vi "setFontFilters.vi"(8 "Error In":errorcluster, 10 "filters":T1 items=["AllFonts"=0, "ScalableFonts"=1, "NonScalableFonts"=2, "MonospacedFonts"=4, "ProportionalFonts"=8], 11 "QFontComboBox In":refnum<class "QFontComboBox.lvclass">) -> (0 "Error Out":errorcluster, 3 "QFontComboBox Out":refnum<class "QFontComboBox.lvclass">)   [LabVIEW 2014, in "QFontComboBox.lvclass"]
doc: "LabVIEW-specific documentation is not yet available. See <b>https://doc.qt.io/qt-5/qfontcombobox.html#setFontFilters</b>"
uses:
  QFontComboBox.lvclass
  FontFilter.ctl
  LQ Core/LQIdentity/LQIdentity.lvclass/LQIdentity.ctl
  LQ Core/LQ Core.lvlib
  LQ Core/LQIdentity/LQIdentity.lvclass
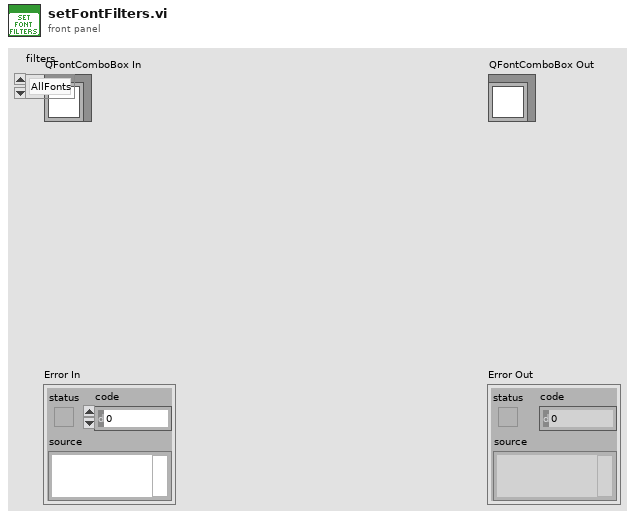
[diagram p1: front panel]
types:
  T1 = typedef "QFontComboBox.lvclass/FontFilter.ctl" = i32
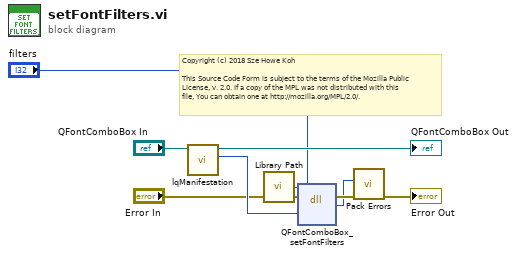
[diagram p0: block diagram]
diagram:
  # "Copyright (c) 2018 Sze Howe Koh\n\nThis Source Code Form is subject to the terms of the Mozilla Public\nLicense, v. 2.0. If a copy of the MPL was not distributed with this\nfile, You can obtain one at http://mozilla.org/MPL/2.0/."
  n1 = call "lqManifestation.vi"("LQIdentity in"="QFontComboBox In") -> ("Manifestation"=w6:u64, "LQIdentity out"=→"QFontComboBox Out":refnum<class "QFontComboBox.lvclass">)  [unwired: 9 in]
  n2 = call "Library Path.vi"() -> ("Library Path"=w7:path)
  n3 = dll-call lib="?" fn="QFontComboBox_setFontFilters"(path in=w7, error in="Error In", "_instance"=w6, "filters"="filters") -> (error out=w4:errorcluster, w2:i32)  [unwired: 3 in, 1 out]
  n4 = call "Pack Errors.vi"("Error In"=w4, "Error Code"=w2) -> ("Error Out"=→"Error Out":errorcluster)  [unwired: 9 in]
